vi "adityam_error_detect.vi"(4 "error in (no error)":errorcluster, 6 "key bit sequence":u8[](array[numeric]), 7 "input bit sequence":u8[](array[numeric])) -> (0 "error out":errorcluster, 3 "bit-error rate":dbl)   [LabVIEW 2026]
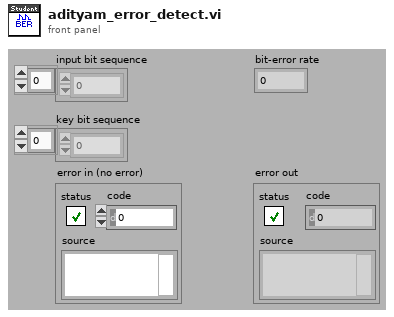
[diagram p1: front panel]
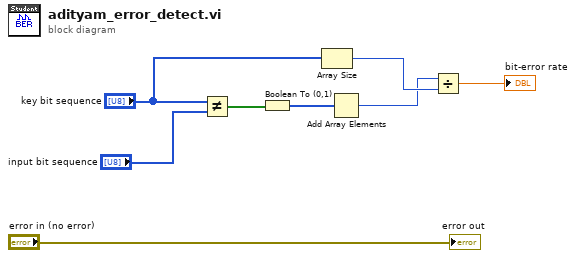
[diagram p0: block diagram]
diagram:
  n1 = Not Equal?(x="key bit sequence", y="input bit sequence") -> (x != y?=w6:bool[])
  n2 = Boolean To (0,1)(Boolean=w6) -> (0, 1=w5:i16[])
  n3 = Array Size(array="key bit sequence") -> (size(s)=w3:i32)
  n4 = Add Array Elements(numeric array=w5) -> (sum=w2:i16)
  n5 = Divide(x=w2, y=w3) -> (x/y=→"bit-error rate":dbl)
  "error out" <- "error in (no error)"
